vi "get default imu config.vi"(8 "error in (no error)":errorcluster) -> (0 "error out":errorcluster, 3 "function return":u32)   [LabVIEW 2014, in "test_IMU.lvlib"]
doc: "imu_config_t get_default_imu_config();"
uses:
  <userlib>/test_IMU/test_IMU.lvlib
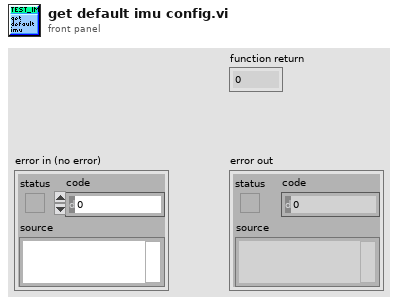
[diagram p1: front panel]
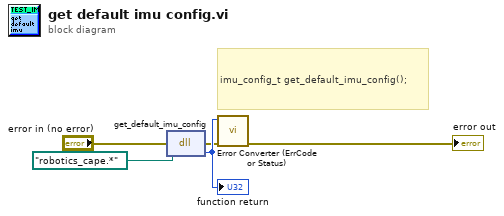
[diagram p0: block diagram]
diagram:
  # "imu_config_t get_default_imu_config();"
  n1 = dll-call lib="C:/Users/ktalke/Documents/Updated Header File/6.18.16/Compiled SO -schroot/robotics_cape.so" fn="get_default_imu_config"(path in=path "robotics_cape.*", error in="error in (no error)") -> (error out=w3:errorcluster, "return type"=w5:u32)  [unwired: 1 in, 1 out]
  "function return" <- w5
  n2 = call <userlib>:"Error Converter (ErrCode or Status).vi"("error in (no error)"=w3, "error code"=w5) -> ("error out"=→"error out":errorcluster)  [unwired: 9 in]
